vi "Home Reference.vi"(8 "Error in":errorcluster, 11 "INL DNL Test in":refnum<class "INL DNL Test.lvclass">) -> (0 "Error out":errorcluster, 1 "Home Ref":refnum<vi>, 2 "VI Ref":refnum<vi>, 3 "INL DNL Test out":refnum<class "INL DNL Test.lvclass">)   [LabVIEW 2020, in "INL DNL Test.lvclass"]
doc: "Runs the home page asynchronously."
uses:
  INL DNL Test.lvclass
  Home Page.vi
  INL DNL Test.lvclass/INL DNL Test.ctl
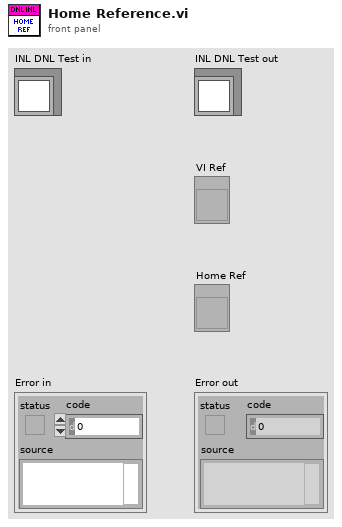
[diagram p1: front panel]
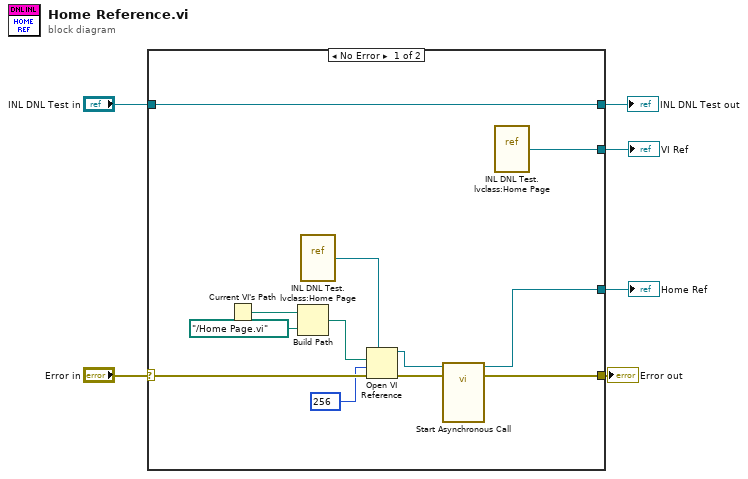
[diagram p0: block diagram]
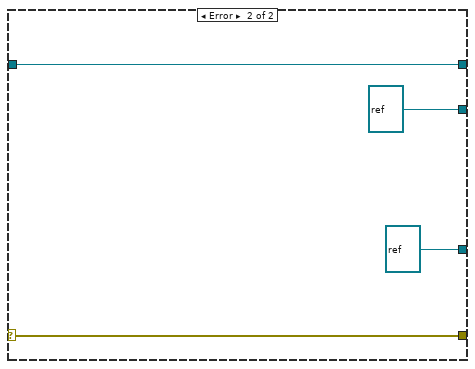
[diagram p2: hidden frame]
diagram:
  n1 = case shown="No Error" "Error in" {
    selector: "Error in" -> [w16 w22]
    tunnel: [w9 w22] -> w5
    tunnel: [w18 w21] -> w3
    tunnel: "INL DNL Test in" -> [w18 w21]
    tunnel: [w17 refnum<vi> refnum] -> w2
    tunnel: [w8 refnum<vi> refnum] -> w1
    frame No Error {
      n2 = Current VI's Path() -> (path=w15:path)
      n3 = Build Path(base path=w15, name or relative path=path "../Home Page.vi") -> (appended path=w13:path)
      n4 = vi-ref "INL DNL Test.lvclass:Home Page.vi"() -> (w12:refnum<vi>)
      n5 = Open VI Reference(type specifier VI Refnum (for type only)=w12, vi path=w13, options=256, error in (no error)=w16) -> (vi reference=w11:refnum<vi>, error out=w10:errorcluster)  [unwired: 2 in]
      n6 = call-by-ref "Start Asynchronous Call"(reference=w11, error in=w10) -> (reference out=w8:refnum<vi>, error out=w9:errorcluster)  [unwired: 15 in, 1 out]
      n7 = vi-ref "INL DNL Test.lvclass:Home Page.vi"() -> (w17:refnum<vi>)
    }
    frame Error {
    }
  }
  "Error out" <- w5
  "INL DNL Test out" <- w3
  "VI Ref" <- w2
  "Home Ref" <- w1
